vi "PCO_CloseCamera.vi"(3 "error in (no error)":errorcluster, 4 "Handle":u64) -> (0 "error out":errorcluster, 1 "Handle Out (success:0, otherwise input)":u32, 2 "return type":u32 format="%x")   [LabVIEW 2011]
uses:
  SC2_Cam64.dll
panel:
  # "A00A3002:not open"
  # "136660040"
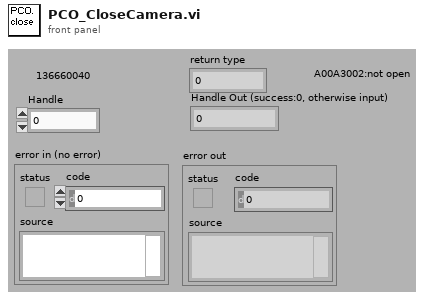
[diagram p1: front panel]
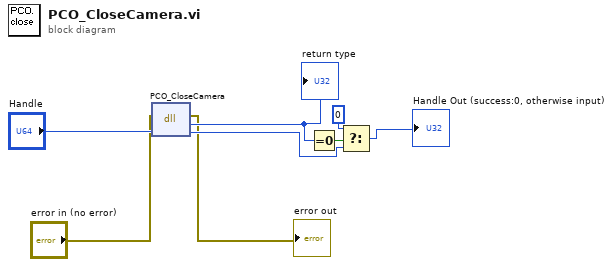
[diagram p0: block diagram]
diagram:
  n1 = dll-call lib="C:/Program Files/colibri/Drivers/PCO.Camera/SC2_Cam*.*" fn="PCO_CloseCamera"(error in="error in (no error)", "Handle"="Handle") -> (error out=→"error out":errorcluster, "return type"=w6:u32, "Handle"=w4:u64)  [unwired: 2 in, 1 out]
  "return type" <- w6
  n2 = Equal To 0?(x=w6) -> (x = 0?=w7:bool)
  n3 = Select(t=u32 0 ("Handle Out"), s=w7, f=w4) -> (s? t:f=→"Handle Out (success:0, otherwise input)":u64)
